vi "Configure CONTFAIL.vi"(0 "VISA resource name":refnum<visa-resource-name>, 5 "CONTFAIL":bool=TRUE, 7 "Configuration Query":bool=TRUE, 11 "error in (no error)":errorcluster) -> (4 "VISA resource name out":refnum<visa-resource-name>, 6 "Query Output":string="\r\n", 8 "Error Message":string, 10 "Error Code":i32, 15 "error out":errorcluster)   [LabVIEW 2010, in "VITREK V7X.lvlib"]
doc: "Configures or Query the <b>Continue sequence on failure</b> setting (0 = no, 1 = yes).\n\n<b>Note:</b> please refer to the instrument manual for the <b>Continue sequence on failure</b> setting specification."
uses:
  VITREK V7X.lvlib
panel:
  # "Yes\n\nNo"
  # "Yes\n\nNo"
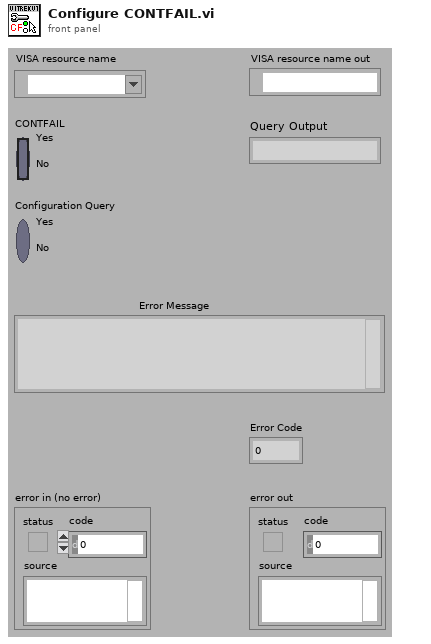
[diagram p1: front panel]
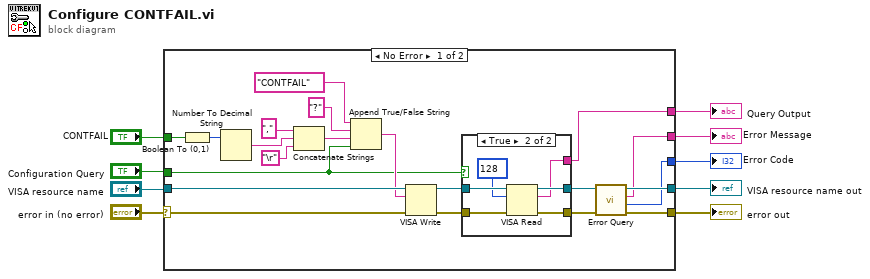
[diagram p0: block diagram]
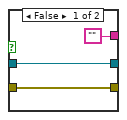
[diagram p2: hidden frame]
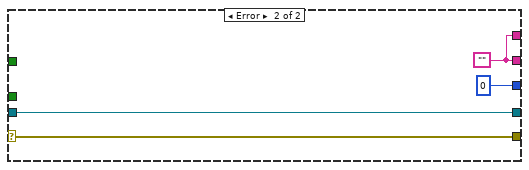
[diagram p3: hidden frame]
diagram:
  n1 = case shown="No Error" "error in (no error)" {
    selector: "error in (no error)" -> [w19 w42]
    tunnel: "VISA resource name" -> [w30 w43]
    tunnel: "Configuration Query" -> [w26 _]
    tunnel: [w24 w41] -> w7
    tunnel: [w21 w43] -> w6
    tunnel: [w20 w42] -> w5
    tunnel: "CONTFAIL" -> [w15 _]
    tunnel: [w12 w41] -> w2
    tunnel: [w11 0 ("Error Code")] -> w1
    frame No Error {
      n2 = Boolean To (0,1)(Boolean=w15) -> (0, 1=w14:i16)
      n3 = Number To Decimal String(number=w14) -> (decimal integer string=w13:string)  [unwired: 1 in]
      n4 = Concatenate Strings(",", w13, "\r") -> (w16:string)
      n5 = Append True/False String(1:w26, 2:w16, 3:"?", 4:"CONTFAIL" ("command")) -> (0:w28:string)
      n6 = VISA Write(VISA resource name=w30, write buffer=w28, error in (no error)=w19) -> (VISA resource name out=w27:refnum<visa-resource-name>, error out=w25:errorcluster)  [unwired: 1 out]
      n7 = case shown="True" w26 {
        tunnel: w27 -> [w33 w37]
        tunnel: [w33 w35] -> w23
        tunnel: w25 -> [w32 w38]
        tunnel: [w32 w39] -> w22
        tunnel: ["" w34] -> w24
        frame False {
        }
        frame True {
          n8 = VISA Read(VISA resource name=w37, byte count=u32 128, error in (no error)=w38) -> (VISA resource name out=w35:refnum<visa-resource-name>, read buffer=w34:string, error out=w39:errorcluster)  [unwired: 1 out]
        }
      }
      n9 = call "Error Query.vi"("error in (no error)"=w22, "VISA resource name"=w23) -> ("error out"=w20:errorcluster, "Error Code"=w11:i32, "Error Message"=w12:string, "VISA resource name out"=w21:refnum<visa-resource-name>)  [unwired: 6 in]
    }
    frame Error {
      w41 = ""
    }
  }
  "VISA resource name out" <- w6
  "error out" <- w5
  "Query Output" <- w7
  "Error Code" <- w1
  "Error Message" <- w2
